vi "TEX_DIM.vi"() -> (0 "TEX_DIM":i16=64)   [LabVIEW 2020]
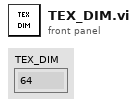
[diagram p1: front panel]
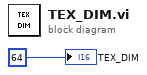
[diagram p0: block diagram]
diagram:
  "TEX_DIM" <- i16 64
